vi "Shutter and DMD OG_Old.vi"(4 "PFI 0 digital clock frequency":dbl, 5 "sCMOS fps":dbl, 6 "OG repitation":dbl, 7 "Objective 线性减速 时间（s）":dbl, 8 "Objective volet 线性减速 时间（s）":dbl, 9 "Objective 刺激steps 时间（s）":dbl, 10 "Objective 线性加速 时间（s）":dbl) -> (2 "DMD OG digital output":bool[](array[boolean]), 3 "Shutter OG digital output":bool[](array[boolean]))   [LabVIEW 2012]
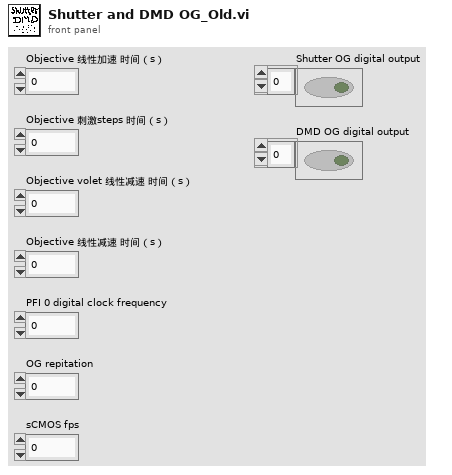
[diagram p1: front panel]
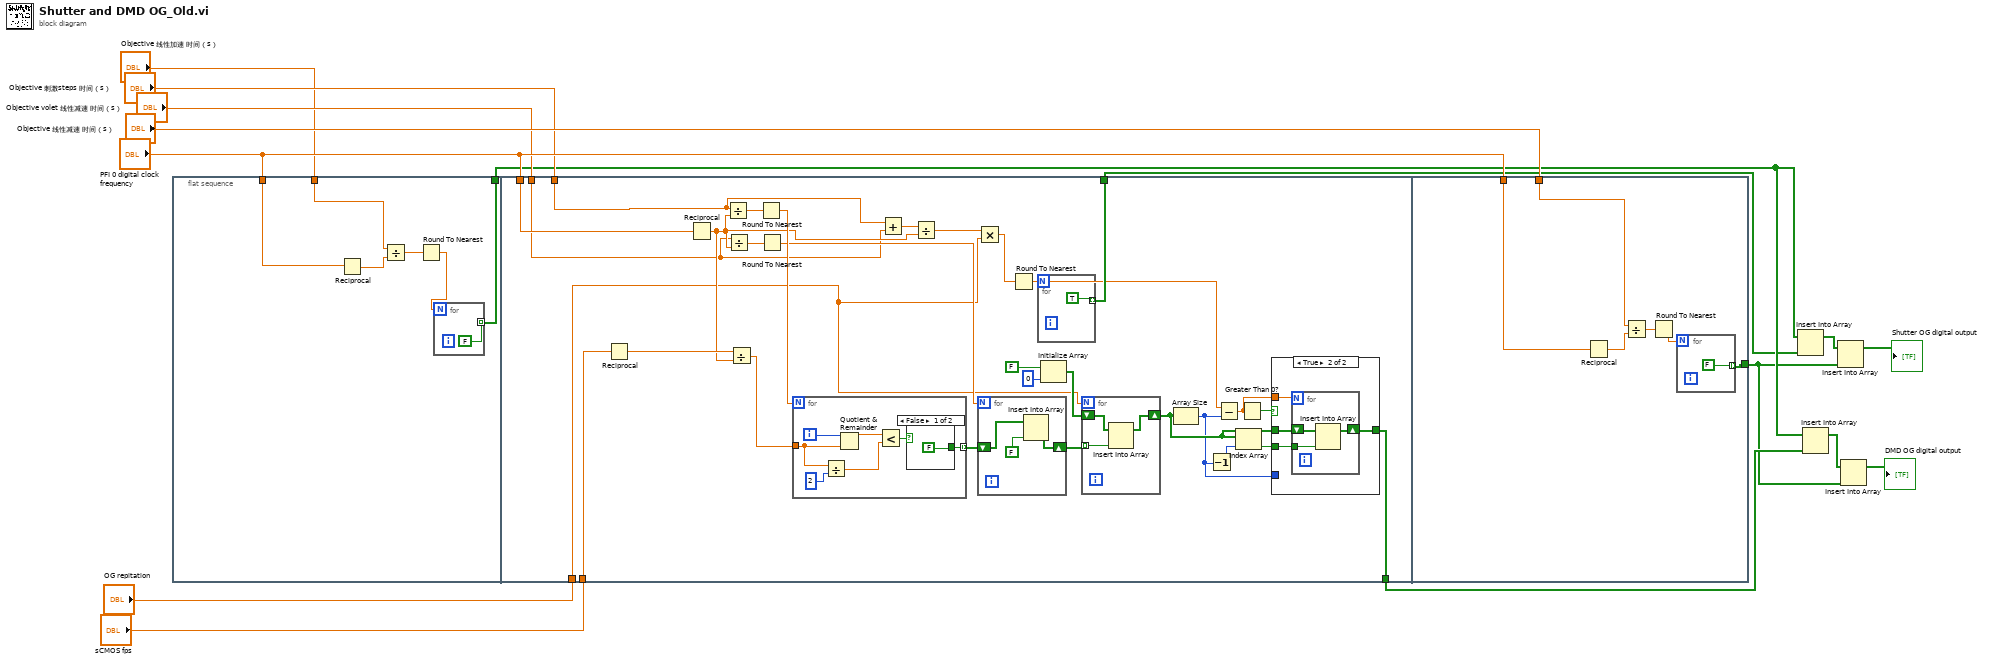
[diagram p0: block diagram]
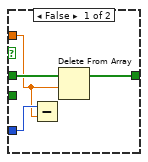
[diagram p2: hidden frame]
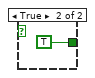
[diagram p3: hidden frame]
diagram:
  n1 = flat-sequence {
    tunnel: [w18] -> w5
    tunnel: "Objective 线性加速 时间（s）" -> [w17]
    tunnel: "PFI 0 digital clock frequency" -> [w16]
    tunnel: [w50] -> w1
    tunnel: [w28] -> w7
    tunnel: "Objective 刺激steps 时间（s）" -> [w27]
    tunnel: "PFI 0 digital clock frequency" -> [w26]
    tunnel: "Objective volet 线性减速 时间（s）" -> [w25]
    tunnel: "OG repitation" -> [w24]
    tunnel: "sCMOS fps" -> [w23]
    tunnel: [w81] -> w4
    tunnel: "Objective 线性减速 时间（s）" -> [w80]
    tunnel: "PFI 0 digital clock frequency" -> [w79]
    frame #0 {
      n2 = Reciprocal(x=w16) -> (1/x=w21:dbl)
      n3 = Divide(x=w17, y=w21) -> (x/y=w20:dbl)
      n4 = Round To Nearest(number=w20) -> (nearest integer value=w19:dbl)
      n5 = for {
        N: w19 -> [_]
        tunnel: [FALSE] -> w18 mode=indexing
      }
    }
    frame #1 {
      n6 = Reciprocal(x=w23) -> (1/x=w47:dbl)
      n7 = Reciprocal(x=w26) -> (1/x=w38:dbl)
      n8 = Divide(x=w27, y=w38) -> (x/y=w49:dbl)
      n9 = Divide(x=w25, y=w38) -> (x/y=w51:dbl)
      n10 = Divide(x=w47, y=w38) -> (x/y=w46:dbl)
      n11 = Round To Nearest(number=w49) -> (nearest integer value=w48:dbl)
      n12 = Round To Nearest(number=w51) -> (nearest integer value=w45:dbl)
      n13 = for {
        N: w48 -> [_]
        tunnel: w46 -> [w74]
        tunnel: [w69] -> w44 mode=indexing
        i -> [w75]
        n14 = Divide(x=w74, y=2) -> (x/y=w71:dbl)
        n15 = Quotient & Remainder(x=w75, y=w74) -> (x-y*floor(x/y)=w72:dbl)  [unwired: 1 out]
        n16 = Less?(x=w72, y=w71) -> (x < y?=w70:bool)
        n17 = case shown="False" w70 {
          tunnel: [FALSE TRUE] -> w69
          frame False {
          }
          frame True {
          }
        }
      }
      n18 = Add(x=w27, y=w25) -> (x+y=w39:dbl)
      n19 = Divide(x=w39, y=w38) -> (x/y=w37:dbl)
      n20 = Multiply(x=w37, y=w24) -> (x*y=w36:dbl)
      n21 = for {
        N: w45 -> [_]
        shift-right: [w66] -> w43
        shift-left: w44 -> [w67]
        n22 = Insert Into Array(array=w67, new element=FALSE) -> (w66:bool[])  [unwired: 1 in]
      }
      n23 = Round To Nearest(number=w36) -> (nearest integer value=w31:dbl)
      n24 = for {
        N: w31 -> [_]
        tunnel: [TRUE] -> w50 mode=indexing
      }
      n25 = Initialize Array(FALSE, 0 ("维数大小")) -> (w40:bool[])
      n26 = for {
        N: w24 -> [_]
        tunnel: w43 -> [w65] mode=indexing
        shift-right: [w63] -> w33
        shift-left: w40 -> [w64]
        n27 = Insert Into Array(array=w64, new element=w65) -> (w63:bool[])  [unwired: 1 in]
      }
      n28 = Array Size(array=w33) -> (size(s)=w29:i32)
      n29 = Decrement(x=w29) -> (x-1=w34:i32)
      n30 = Subtract(x=w31, y=w29) -> (x-y=w30:dbl)
      n31 = Index Array(array=w33, index=w34) -> (element=w32:bool)
      n32 = Greater Than 0?(x=w30) -> (x > 0?=w35:bool)
      n33 = case shown="True" w35 {
        tunnel: w33 -> [w55 w59]
        tunnel: w32 -> [_ w58]
        tunnel: w30 -> [w52 w57]
        tunnel: [w54 w56] -> w28
        tunnel: w29 -> [w53 _]
        frame False {
          n34 = Subtract(x=w53, y=w52) -> ()  [unwired: 1 out]
          n35 = Delete From Array(array=w55, length=w52) -> (array with subset deleted=w54:bool[])  [unwired: 1 in, 1 out]
        }
        frame True {
          n36 = for {
            N: w57 -> [_]
            tunnel: w58 -> [w61]
            shift-right: [w60] -> w56
            shift-left: w59 -> [w62]
            n37 = Insert Into Array(array=w62, new element=w61) -> (w60:bool[])  [unwired: 1 in]
          }
        }
      }
    }
    frame #2 {
      n38 = Reciprocal(x=w79) -> (1/x=w84:dbl)
      n39 = Divide(x=w80, y=w84) -> (x/y=w83:dbl)
      n40 = Round To Nearest(number=w83) -> (nearest integer value=w82:dbl)
      n41 = for {
        N: w82 -> [_]
        tunnel: [FALSE] -> w81 mode=indexing
      }
    }
  }
  n42 = Insert Into Array(array=w5, new element=w1) -> (w2:bool[])  [unwired: 1 in]
  n43 = Insert Into Array(array=w5, new element=w7) -> (w6:bool[])  [unwired: 1 in]
  n44 = Insert Into Array(array=w2, new element=w4) -> (→"Shutter OG digital output":bool[])  [unwired: 1 in]
  n45 = Insert Into Array(array=w6, new element=w4) -> (→"DMD OG digital output":bool[])  [unwired: 1 in]
